vi "2024_day09_Task01.vi"() -> ()   [LabVIEW 2023]
uses:
  <userlib>/_OpenG.lib/array/array.llb/Search 1D Array (I32)__ogtk.vi
  <userlib>/_OpenG.lib/array/array.llb/Delete Elements from 1D Array (I32)__ogtk.vi
  <userlib>/_OpenG.lib/string/string.llb/openg_string.lvlib
  <userlib>/_OpenG.lib/array/array.llb/openg_array.lvlib
panel:
  out "Result - Task 1":i64
  in  "Switch":bool caption="Ex. Data  vs.  User Data"
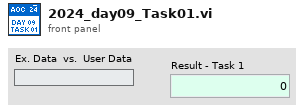
[diagram p1: front panel]
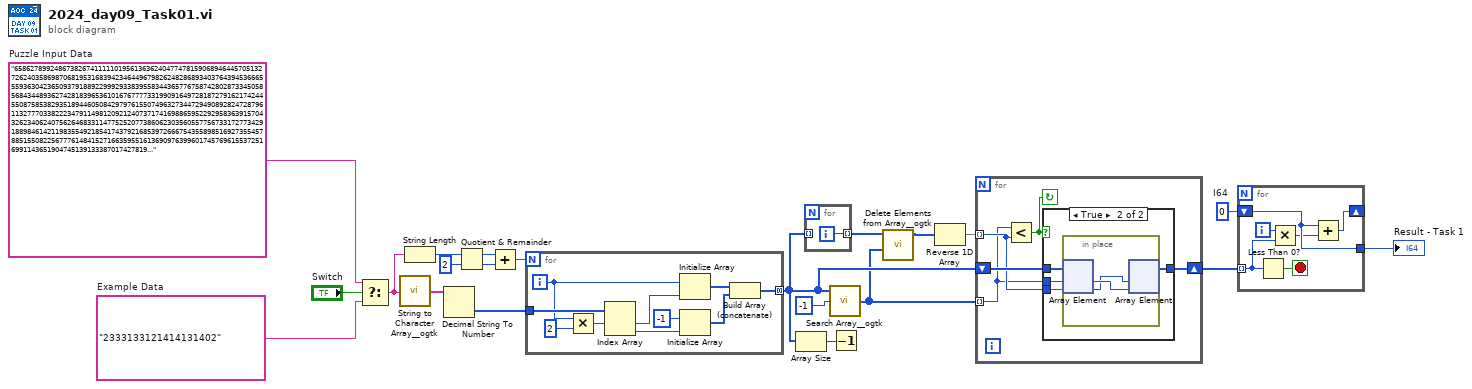
[diagram p0: block diagram]
diagram:
  w2 = i64 0  # I64
  w19 = "658627899248673826741111101956136362404774781590689464457051327262403586987068195316839423464496798262482868934037643945366655593630423650937918892299929338395583443657767587428028733450585684344893627428183965361016767777331990916497281872791621742445508758538293518944605084297976155074963273447294908928247287961132777033822234791149812092124073717416988659522929583639157043262340624075626468331147752520773860623035605577567331727734291889846142119835549218541743792168539726667543558985169273554578851550822567776148415271663595516136909763996017457696155372516991143651904745139133387017427819..."  # Puzzle Input Data
  w20 = "2333133121414131402"  # Example Data
  n1 = Select(t=w19, s="Switch", f=w20) -> (s? t:f=w17:string)
  n2 = call <userlib>:"String to Character Array__ogtk.vi"("Input String"=w17) -> ("Character Array"=w18:string[])
  n3 = String Length(string=w17) -> (length=w16:i32)
  n4 = Decimal String To Number(string=w18) -> (number=w13:i32[])  [unwired: 2 in, 1 out]
  n5 = Quotient & Remainder(x=w16, y=2) -> (x-y*floor(x/y)=w11:i32, floor(x/y)=w14:i32)
  n6 = Add(x=w11, y=w14) -> (x+y=w12:i32)
  n7 = for {
    N: w12 -> [_]
    tunnel: [w28] -> w7 mode=concatenating
    tunnel: w13 -> [w27]
    i -> [w24]
    n8 = Multiply(x=w24, y=2) -> (x*y=w23:i32)
    n9 = Index Array(array=w27, index #1=w23) -> (element #1=w26:i32, element #2=w25:i32)  [unwired: 1 in]
    n10 = Initialize Array(w24, w26) -> (w31:i32[])
    n11 = Initialize Array(-1 ("element"), w25) -> (w30:i32[])
    n12 = Build Array (concatenate)(w31, w30) -> (w28:i32[])
  }
  n13 = Array Size(array=w7) -> (size(s)=w9:i32)
  n14 = for {
    tunnel: [w32] -> w6 mode=indexing
    tunnel: w7 -> [_] mode=indexing
    i -> [w32]
  }
  n15 = call-poly <userlib>:"Search Array__ogtk.vi"("Array"=w7, "Element Data"=-1) -> ("Indices of Elements"=w5:i32[])  [unwired: 7 in]
  n16 = Decrement(x=w9) -> ()  [unwired: 1 out]
  n17 = call-poly <userlib>:"Delete Elements from Array__ogtk.vi"("indices"=w5, "array"=w6) -> ("array w/ subset deleted"=w4:i32[])  [unwired: 8 in, 1 out]
  n18 = Reverse 1D Array(array=w4) -> (reversed array=w3:i32[])
  n19 = for {
    tunnel: w5 -> [w34] mode=indexing
    shift-right: [w36] -> w8
    shift-left: w7 -> [w37]
    tunnel: w3 -> [w35] mode=indexing
    stop <- w33 continue-if-true
    n20 = Less?(x=w34, y=w35) -> (x < y?=w33:bool)
    n21 = case shown="True" w33 {
      tunnel: w37 -> [w38 w42]
      tunnel: [w38 w41] -> w36
      tunnel: w35 -> [_ w40]
      tunnel: w34 -> [_ w39]
      frame False {
      }
      frame True {
        n22 = in-place {
          n23 = in-place-array #1(w42, w39, w40) -> (w44:i32, w43:i32)
          n24 = in-place-array #1(w43, w44) -> (w41:i32[])  [unwired: 2 out]
        }
      }
    }
  }
  n25 = for {
    tunnel: w8 -> [w49] mode=indexing
    shift-right: [w45] -> _
    shift-left: w2 -> [w47]
    tunnel: [w47] -> w1
    i -> [w48]
    stop <- w50 stop-if-true
    n26 = Less Than 0?(x=w49) -> (x < 0?=w50:bool)
    n27 = Multiply(x=w48, y=w49) -> (x*y=w46:i32)
    n28 = Add(x=w47, y=w46) -> (x+y=w45:i64)
  }
  "Result - Task 1" <- w1
